vi "Get Data.vi"(8 "error in":errorcluster, 11 "Meerstetter TEC in":refnum<class "Meerstetter TEC.lvclass">) -> (0 "error out":errorcluster, 2 "DataOut":refnum<class "Data.lvclass">, 3 "Meerstetter TEC out":refnum<class "Meerstetter TEC.lvclass">)   [LabVIEW 2014, in "Meerstetter Lib.lvlib" / "Meerstetter TEC.lvclass"]
uses:
  Meerstetter TEC.lvclass
  reusable/Data/Data.lvclass
  Data/mTEC Data.lvclass
  Configurable Device/Configurable Device.lvclass/Configurable Device.ctl
  Data/mTEC Data.lvclass/mTEC Data.ctl
  reusable/Data/Data.lvclass/Data.ctl
  Configurable Device/Read ID.vi
  Data/Write Tobj.vi
  Data/Write Tsink.vi
  Data/Write Vout.vi
  reusable/Data/Write Data ID.vi
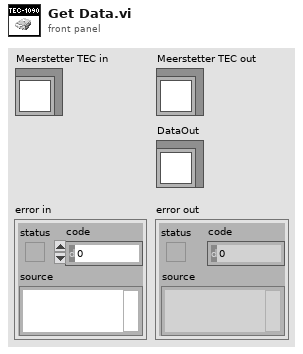
[diagram p1: front panel]
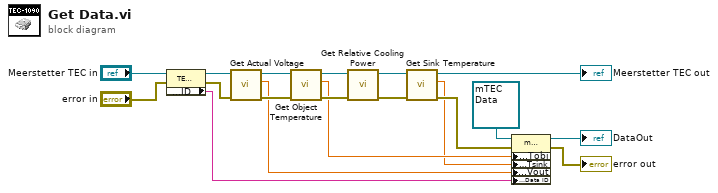
[diagram p0: block diagram]
diagram:
  n1 = property class="TEC 1090"(reference="Meerstetter TEC in", error in="error in") -> (reference out=w3:refnum<class "Meerstetter TEC.lvclass">, error out=w1:errorcluster, "Accessors:ID"=w4:string)
  n2 = call "Get Actual Voltage.vi"("error in"=w1, "TEC 1090 in"=w3) -> ("error out"=w16:errorcluster, "Number"=w9:sgl, "TEC 1090 out"=w19:refnum<class "Meerstetter TEC.lvclass">)  [unwired: 7 in]
  n3 = call "Get Object Temperature.vi"("error in"=w16, "TEC 1090 in"=w19) -> ("error out"=w17:errorcluster, "Number"=w11:sgl, "TEC 1090 out"=w18:refnum<class "Meerstetter TEC.lvclass">)  [unwired: 7 in]
  n4 = call "Get Relative Cooling Power.vi"("error in"=w17, "TEC 1090 in"=w18) -> ("error out"=w14:errorcluster, "TEC 1090 out"=w15:refnum<class "Meerstetter TEC.lvclass">)  [unwired: 7 in, 1 out]
  n5 = call "Get Sink Temperature.vi"("error in"=w14, "TEC 1090 in"=w15) -> ("error out"=w12:errorcluster, "Number"=w10:sgl, "TEC 1090 out"=→"Meerstetter TEC out":refnum<class "Meerstetter TEC.lvclass">)  [unwired: 7 in]
  n6 = property class="mTEC Data.lvclass"(reference=refnum<class "mTEC Data.lvclass"> refnum ("Meerstetter Lib.lvlib:mTEC Data.lvclass"), error in=w12, "Accessors:Tobj"=w11, "Accessors:Tsink"=w10, "Accessors:Vout"=w9, "Accessors:Data ID"=w4) -> (reference out=→"DataOut":refnum<class "mTEC Data.lvclass">, error out=→"error out":errorcluster)
